vi "Translate Settings.vi"(0 "data":u8[](array[numeric]), 1 "Step time(uS)":dbl[](array[numeric]), 11 "Command mode":enum16{"CW Frequency", "Sweep Frequency"}(ring)) -> (6 "Actual settings":T1 {"CWFreq(GHz)" format="%#_12g"; "RiseStepDwellTime(uS)" format="%#_12g"; "FallStepDwellTime(uS)" format="%#_12g"; "RiseTime(mS)" format="%#_14g"; "FallTime(mS)" format="%#_14g"; "StartFreq(GHz)" format="%#_12g"; "StopFreq(GHz)" format="%#_12g"; "RiseStepSize(Hz)" format="%#_12g"; "FallStepSize(Hz)" format="%#_12g"; "Rise#Steps" format="%#_12g"; "Fall#Steps" format="%#_12g"})   [LabVIEW 2021]
panel:
  out "FallTime(mS)":dbl format="%#_14g"
  out "RiseTime(mS)":dbl format="%#_14g"
  out "Fall#Steps":dbl format="%#_12g"
  out "Rise#Steps":dbl format="%#_12g"
  out "FallStepDwellTime(uS)":dbl format="%#_12g"
  out "RiseStepDwellTime(uS)":dbl format="%#_12g"
  out "FallStepSize(Hz)":dbl format="%#_12g"
  out "RiseStepSize(Hz)":dbl format="%#_12g"
  out "StopFreq(GHz)":dbl format="%#_12g"
  out "StartFreq(GHz)":dbl format="%#_12g"
  out "CWFreq(GHz)":dbl format="%#_12g"
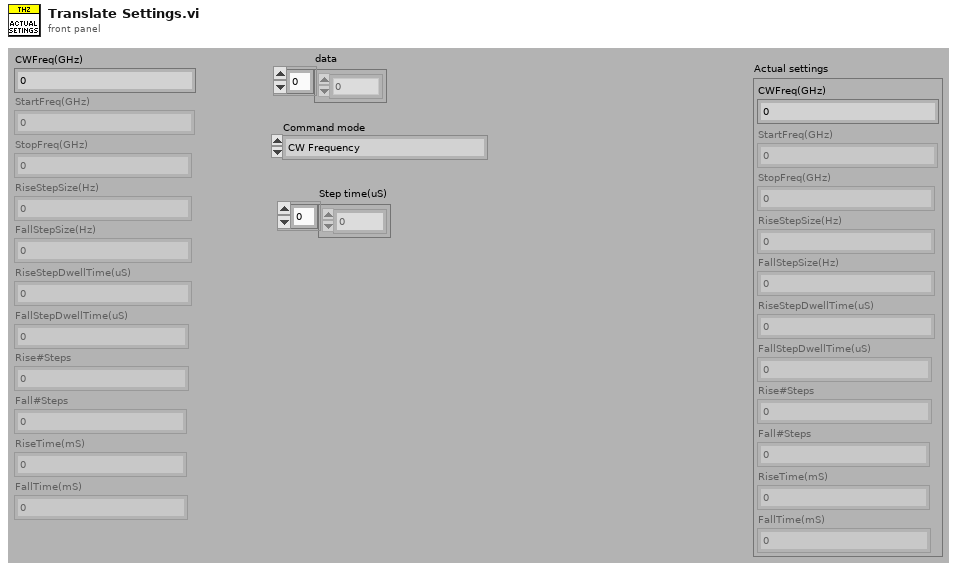
[diagram p1: front panel]
types:
  T1 = cluster{"CWFreq(GHz)":dbl, "StartFreq(GHz)":dbl, "StopFreq(GHz)":dbl, "RiseStepSize(Hz)":dbl, "FallStepSize(Hz)":dbl, "RiseStepDwellTime(uS)":dbl, "FallStepDwellTime(uS)":dbl, "Rise#Steps":dbl, "Fall#Steps":dbl, "RiseTime(mS)":dbl, "FallTime(mS)":dbl}
  T2 = cluster{"CWFreq(GHz) 2":dbl, "StartFreq(GHz) 2":dbl, "StopFreq(GHz) 2":dbl, "RiseStepSize(Hz) 2":dbl, "FallStepSize(Hz) 2":dbl, "RiseStepDwellTime(uS) 2":dbl, "FallStepDwellTime(uS) 2":dbl, "Rise#Steps 2":dbl, "Fall#Steps 2":dbl, "RiseTime(mS) 2":dbl, "FallTime(mS) 2":dbl}
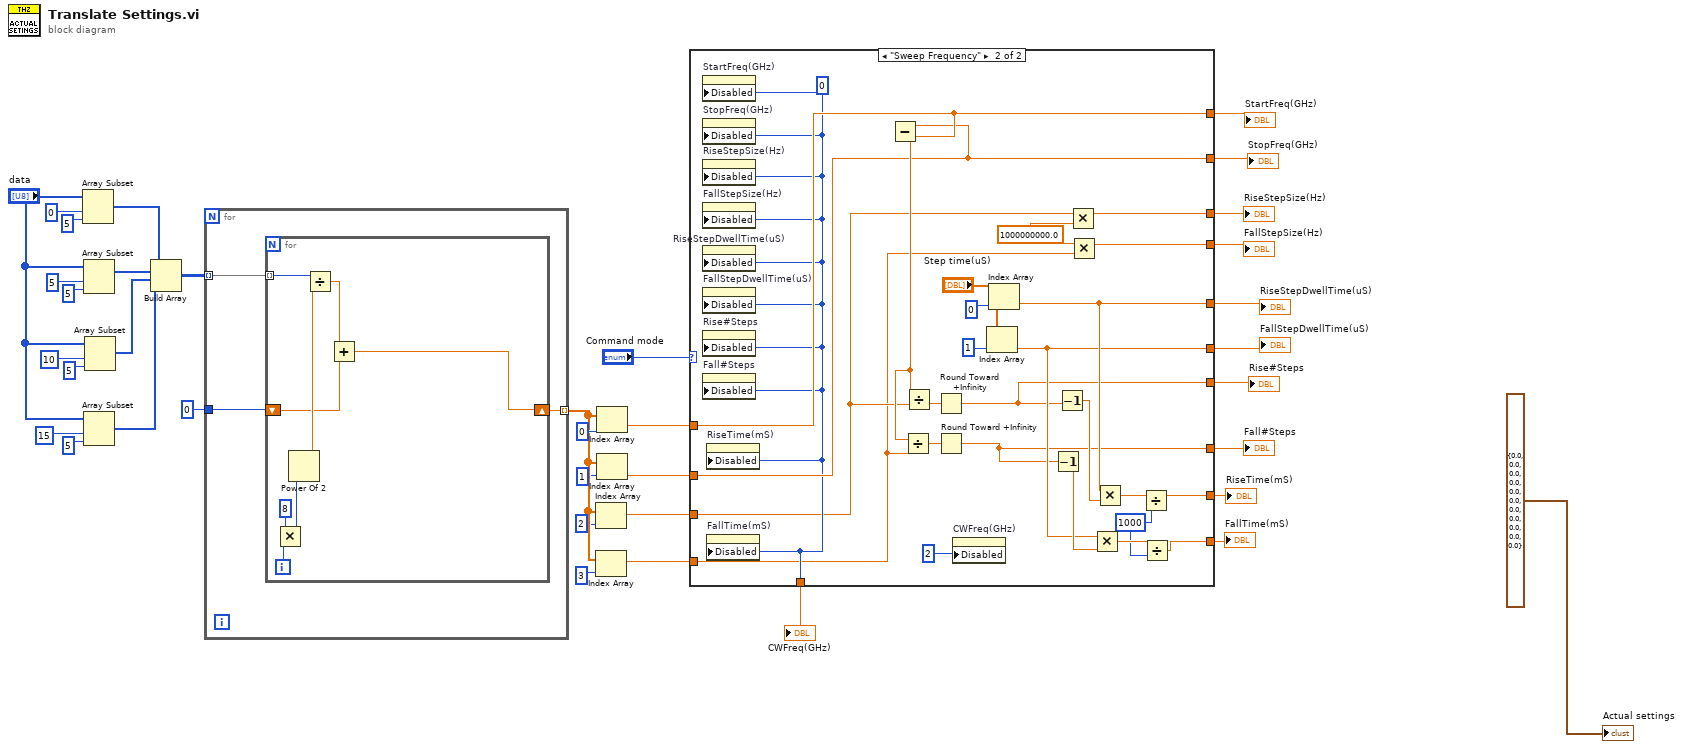
[diagram p0: block diagram]
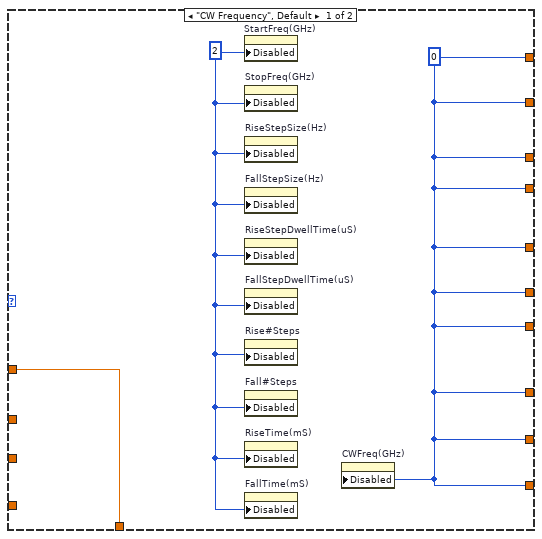
[diagram p2: hidden frame]
diagram:
  n1 = Array Subset(array="data", index=0, length=5) -> (w28:u8[])
  n2 = Array Subset(array="data", index=5, length=5) -> (w27:u8[])
  n3 = Array Subset(array="data", index=15, length=5) -> (w25:u8[])
  n4 = Array Subset(array="data", index=10, length=5) -> (w26:u8[])
  n5 = Build Array(w28, w27, w26, w25) -> (w24:u8[][])
  n6 = for {
    tunnel: w24 -> [w40] mode=indexing
    tunnel: 0 -> [w39]
    tunnel: [w38] -> w21 mode=indexing
    n7 = for {
      tunnel: w40 -> [w45] mode=indexing
      shift-right: [w41] -> w38
      shift-left: w39 -> [w42]
      i -> [w48]
      n8 = Multiply(x=8, y=w48) -> (x*y=w46:i32)
      n9 = Power Of 2(x=w46) -> (2^x=w44:dbl)
      n10 = Divide(x=w45, y=w44) -> (x/y=w43:dbl)
      n11 = Add(x=w43, y=w42) -> (x+y=w41:dbl)
    }
  }
  n12 = Index Array(array=w21, index=2) -> (element=w14:dbl)
  n13 = Index Array(array=w21, index=3) -> (element=w13:dbl)
  n14 = Index Array(array=w21, index=0) -> (element=w16:dbl)
  n15 = Index Array(array=w21, index=1) -> (element=w15:dbl)
  n16 = case shown="\"Sweep Frequency\"" "Command mode" {
    tunnel: w16 -> [w50 w67]
    tunnel: w15 -> [_ w66]
    tunnel: w14 -> [_ w56]
    tunnel: w13 -> [_ w53]
    tunnel: [w49 w69] -> w12
    tunnel: [w49 w68] -> w11
    tunnel: [w49 w60] -> w10
    tunnel: [w49 w59] -> w9
    tunnel: [w49 w67] -> w8
    tunnel: [w49 w66] -> w7
    tunnel: [w49 w55] -> w6
    tunnel: [w49 w54] -> w5
    tunnel: [w49 w65] -> w4
    tunnel: [w49 w64] -> w3
    tunnel: [w50 w63] -> w2
    frame "CW Frequency", Default {
      w51 = 2
      w49 = 0
      n17 = property on="StartFreq(GHz)" class="DigNum (strict)"("Disabled"=w51) -> ()  [unwired: 2 in, 2 out]
      n18 = property on="StopFreq(GHz)" class="DigNum (strict)"("Disabled"=w51) -> ()  [unwired: 2 in, 2 out]
      n19 = property on="RiseStepSize(Hz)" class="DigNum (strict)"("Disabled"=w51) -> ()  [unwired: 2 in, 2 out]
      n20 = property on="FallStepSize(Hz)" class="DigNum (strict)"("Disabled"=w51) -> ()  [unwired: 2 in, 2 out]
      n21 = property on="RiseStepDwellTime(uS)" class="DigNum (strict)"("Disabled"=w51) -> ()  [unwired: 2 in, 2 out]
      n22 = property on="FallStepDwellTime(uS)" class="DigNum (strict)"("Disabled"=w51) -> ()  [unwired: 2 in, 2 out]
      n23 = property on="Rise#Steps" class="DigNum (strict)"("Disabled"=w51) -> ()  [unwired: 2 in, 2 out]
      n24 = property on="Fall#Steps" class="DigNum (strict)"("Disabled"=w51) -> ()  [unwired: 2 in, 2 out]
      n25 = property on="RiseTime(mS)" class="DigNum (strict)"("Disabled"=w51) -> ()  [unwired: 2 in, 2 out]
      n26 = property on="FallTime(mS)" class="DigNum (strict)"("Disabled"=w51) -> ()  [unwired: 2 in, 2 out]
      n27 = property on="CWFreq(GHz)" class="DigNum (strict)"("Disabled"=w49) -> ()  [unwired: 2 in, 2 out]
    }
    frame "Sweep Frequency" {
      w52 = 1000000000.0
      w57 = 1000
      w63 = 0
      n28 = property on="StartFreq(GHz)" class="DigNum (strict)"("Disabled"=w63) -> ()  [unwired: 2 in, 2 out]
      n29 = property on="StopFreq(GHz)" class="DigNum (strict)"("Disabled"=w63) -> ()  [unwired: 2 in, 2 out]
      n30 = property on="RiseStepSize(Hz)" class="DigNum (strict)"("Disabled"=w63) -> ()  [unwired: 2 in, 2 out]
      n31 = property on="FallStepSize(Hz)" class="DigNum (strict)"("Disabled"=w63) -> ()  [unwired: 2 in, 2 out]
      n32 = property on="RiseStepDwellTime(uS)" class="DigNum (strict)"("Disabled"=w63) -> ()  [unwired: 2 in, 2 out]
      n33 = property on="FallStepDwellTime(uS)" class="DigNum (strict)"("Disabled"=w63) -> ()  [unwired: 2 in, 2 out]
      n34 = property on="Rise#Steps" class="DigNum (strict)"("Disabled"=w63) -> ()  [unwired: 2 in, 2 out]
      n35 = property on="Fall#Steps" class="DigNum (strict)"("Disabled"=w63) -> ()  [unwired: 2 in, 2 out]
      n36 = property on="RiseTime(mS)" class="DigNum (strict)"("Disabled"=w63) -> ()  [unwired: 2 in, 2 out]
      n37 = property on="FallTime(mS)" class="DigNum (strict)"("Disabled"=w63) -> ()  [unwired: 2 in, 2 out]
      n38 = Subtract(x=w66, y=w67) -> (x-y=w74:dbl)
      n39 = Divide(x=w74, y=w53) -> (x/y=w72:dbl)
      n40 = Divide(x=w74, y=w56) -> (x/y=w73:dbl)
      n41 = Round Toward +Infinity(x=w73) -> (ceil(x): smallest int >= x=w65:dbl)
      n42 = Round Toward +Infinity(x=w72) -> (ceil(x): smallest int >= x=w64:dbl)
      n43 = property on="CWFreq(GHz)" class="DigNum (strict)"("Disabled"=2) -> ()  [unwired: 2 in, 2 out]
      n44 = Index Array(array="Step time(uS)", index=1) -> (element=w68:dbl)
      n45 = Index Array(array="Step time(uS)", index=0) -> (element=w69:dbl)
      n46 = Decrement(x=w64) -> (x-1=w70:dbl)
      n47 = Decrement(x=w65) -> (x-1=w71:dbl)
      n48 = Multiply(x=w56, y=w52) -> (x*y=w55:dbl)
      n49 = Multiply(x=w52, y=w53) -> (x*y=w54:dbl)
      n50 = Multiply(x=w68, y=w70) -> (x*y=w58:dbl)
      n51 = Multiply(x=w69, y=w71) -> (x*y=w61:dbl)
      n52 = Divide(x=w61, y=w57) -> (x/y=w59:dbl)
      n53 = Divide(x=w58, y=w57) -> (x/y=w60:dbl)
    }
  }
  "RiseStepDwellTime(uS)" <- w12
  "FallStepDwellTime(uS)" <- w11
  "RiseTime(mS)" <- w9
  "FallTime(mS)" <- w10
  "StartFreq(GHz)" <- w8
  "StopFreq(GHz)" <- w7
  "RiseStepSize(Hz)" <- w6
  "FallStepSize(Hz)" <- w5
  "Rise#Steps" <- w4
  "Fall#Steps" <- w3
  "CWFreq(GHz)" <- w2
  "Actual settings" <- T2 {"CWFreq(GHz) 2"=0.0, "StartFreq(GHz) 2"=0.0, "StopFreq(GHz) 2"=0.0, "RiseStepSize(Hz) 2"=0.0, "FallStepSize(Hz) 2"=0.0, "RiseStepDwellTime(uS) 2"=0.0, "FallStepDwellTime(uS) 2"=0.0, "Rise#Steps 2"=0.0, "Fall#Steps 2"=0.0, "RiseTime(mS) 2"=0.0, "FallTime(mS) 2"=0.0} ("Actual settings")
